vi "sub_autocreate_device_and_type_name.vi"(9 "Device_Key in":string) -> (1 "Device_Key out":string)   [LabVIEW 2013, in "daqio minimal.lvlib"]
doc: "This VI will automatically create a Device Key and a Device Type Key based on the current machine's hostname if no existing Keys are present."
uses:
  daqio minimal.lvlib
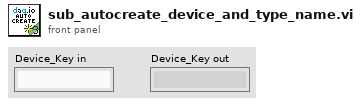
[diagram p1: front panel]
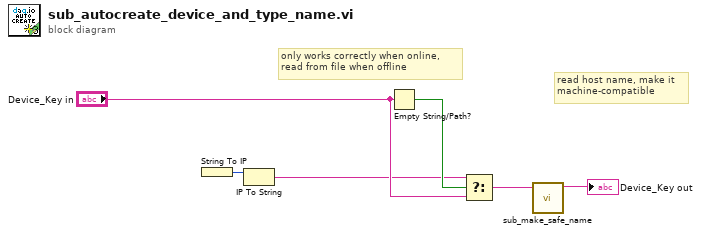
[diagram p0: block diagram]
diagram:
  # "only works correctly when online, \nread from file when offline"
  # "read host name, make it \nmachine-compatible"
  n1 = String To IP() -> (0:w4:u32)  [unwired: 1 in]
  n2 = IP To String(2:w4) -> (0:w3:string)  [unwired: 1 in]
  n3 = Empty String/Path?(string/path="Device_Key in") -> (empty?=w5:bool)
  n4 = Select(t=w3, s=w5, f="Device_Key in") -> (s? t:f=w2:string)
  n5 = call "sub_make_safe_name.vi"("Input String"=w2) -> ("Safe Output String"=→"Device_Key out":string)  [unwired: 10 in]
